vi "Get LogicIO by Label.vi"(8 "error in (no error)":errorcluster, 10 "label":string, 11 "VacuumLine in":refnum<class "VacuumLine.lvclass">) -> (0 "error out":errorcluster, 1 "found":bool, 2 "LogicIO obj":refnum<class "LogicIO.lvclass">, 3 "VacuumLine out":refnum<class "VacuumLine.lvclass">)   [LabVIEW 2016, in "Hardware.lvlib" / "VacuumLine.lvlib" / "VacuumLine.lvclass"]
uses:
  <userlib>/Common Components/Hardware/Abstract System/VacuumLine/VacuumLine/VacuumLine.lvclass
  <userlib>/Common Components/Hardware/LogicIO/LogicIO/LogicIO.lvclass
  <userlib>/Common Components/Hardware/Abstract System/VacuumLine/VacuumLine/VacuumLine.lvclass/VacuumLine.ctl
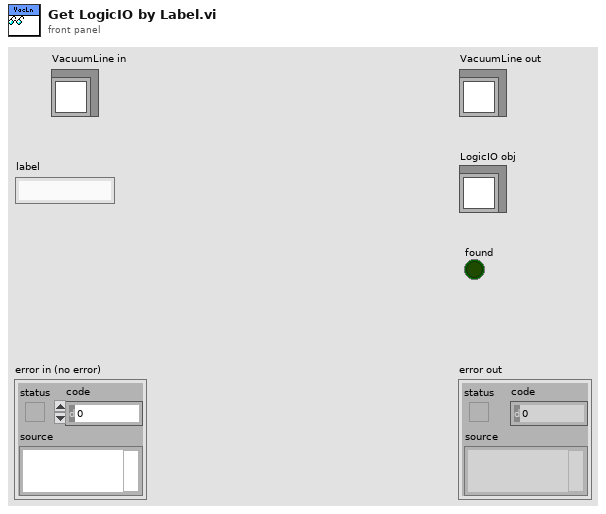
[diagram p1: front panel]
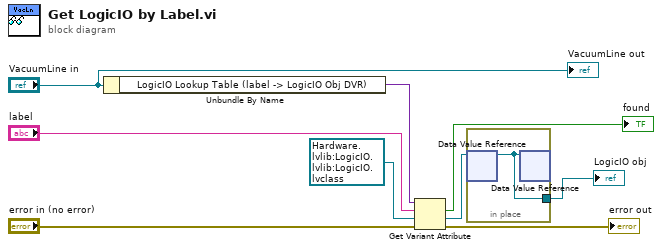
[diagram p0: block diagram]
diagram:
  n1 = Unbundle By Name("VacuumLine in") -> ("LogicIO Lookup Table (label -> LogicIO Obj DVR)"=w8:variant)
  n2 = Get Variant Attribute(Variant=w8, name="label", default value (empty Variant)=refnum<data-value> refnum ("data value reference"), error in="error in (no error)") -> (found=→"found":bool, value=w2:refnum<data-value>, error out=→"error out":errorcluster)  [unwired: 1 out]
  n3 = in-place {
    in-place-border: [w10] -> w1
    n4 = in-place-dvr #1(w2) -> (w10:refnum<class "LogicIO.lvclass">)  [unwired: 1 out]
    n5 = in-place-dvr #1(w10) -> ()  [unwired: 2 out]
  }
  "LogicIO obj" <- w1
  "VacuumLine out" <- "VacuumLine in"
